vi "Read Value.vi"(8 "error in (no error)":errorcluster caption="entrée d'erreur (pas d'erreur)", 11 "DAQmxTaskDOutput en entrée":refnum<class "DAQmxTaskDOutput.lvclass">) -> (0 "error out":errorcluster caption="sortie d'erreur", 1 "data":bool caption="Data", 2 "Data string":string, 3 "DAQmxTaskDOutput en sortie":refnum<class "DAQmxTaskDOutput.lvclass">)   [LabVIEW 2015, in "DAQmxTaskDOutput.lvclass"]
uses:
  DAQmxTaskDOutput.lvclass
  DAQmxTask.lvclass/DAQmxTask.ctl
  <vilib>/DAQmx/read.llb/DAQmx Read (Digital Bool 1Line 1Point).vi
  <vilib>/DAQmx/miscellaneous.llb/DAQmx Fill In Error Info.vi
  DAQmxTask.lvclass
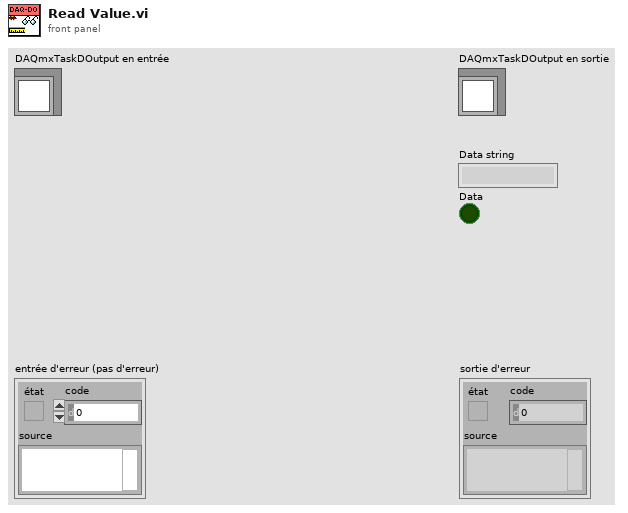
[diagram p1: front panel]
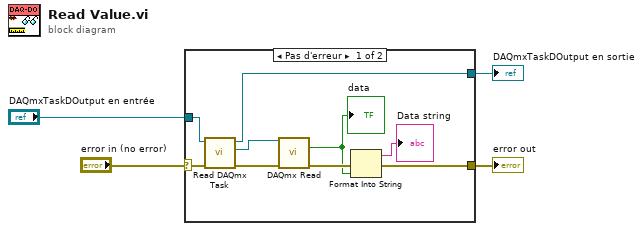
[diagram p0: block diagram]
diagram:
  n1 = case shown="Pas d'erreur" "error in (no error)" {
    selector: "error in (no error)" -> [w13 w15]
    tunnel: [w6 w15] -> w3
    tunnel: [w5 w14] -> w2
    tunnel: "DAQmxTaskDOutput en entrée" -> [w8 w14]
    frame No Error {
      n2 = call "Read DAQmx Task.vi"("error in (no error)"=w13, "DAQmxTask in"=w8) -> ("error out"=w11:errorcluster, "DAQmx Task Name"=w12:refnum<k21>, "DAQmxTask out"=w5:refnum<class "DAQmxTaskDOutput.lvclass">)  [unwired: 7 in]
      n3 = call-poly <vilib>:"DAQmx Read.vi"("task/channels in"=w12, "error in"=w11) -> ("data"=w9:bool, "error out"=w10:errorcluster)  [unwired: 11 in, 1 out]
      "data" <- w9
      n4 = Format Into String(error in=w10, w9) -> (resulting string=→"Data string":string, error out=w6:errorcluster)  [unwired: 2 in]
    }
    frame Error {
    }
  }
  "error out" <- w3
  "DAQmxTaskDOutput en sortie" <- w2
